vi "Test Magnet.vi"(8 "error in (no error)":errorcluster, 11 "Instrument.Cryostat in":refnum<class "Instrument.Cryostat.lvclass">) -> (0 "error out":errorcluster, 3 "Instrument.Cryostat out":refnum<class "Instrument.Cryostat.lvclass">)   [LabVIEW 2016]
uses:
  lvsrc/Instrument Types/Cryostat/Instrument.Cryostat.lvclass
  <vilib>/addons/_JKI Toolkits/Caraya/classes/Assert/Assert.lvclass
  <vilib>/addons/_JKI Toolkits/Caraya/classes/Test/Test.lvclass
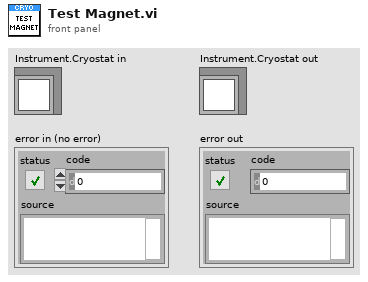
[diagram p1: front panel]
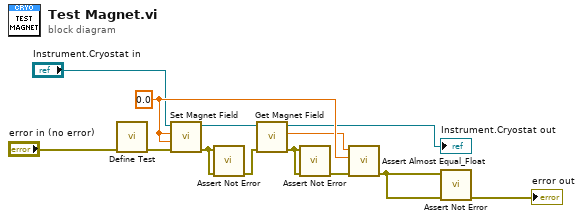
[diagram p0: block diagram]
diagram:
  w8 = 0.0 ("Angle (°)")
  n1 = call <vilib>:"Define Test.vi"("error in (no error)"="error in (no error)") -> ("error out"=w2:errorcluster)  [unwired: 10 in]
  n2 = call-dynamic "Set Magnet Field.vi"("error in (no error)"=w2, "Target Rate (T/min)"=w8, "Target Field (T)"=w8, "Instrument.Cryostat in"="Instrument.Cryostat in") -> ("error out"=w9:errorcluster, "Instrument.Cryostat out"=w6:refnum<class "Instrument.Cryostat.lvclass">)  [unwired: 6 in]
  n3 = call <vilib>:"Assert Not Error.vi"("error in (no error)"=w9, "Not Error?"=w9) -> ("error out"=w10:errorcluster)  [unwired: 9 in]
  n4 = call-dynamic "Get Magnet Field.vi"("error in (no error)"=w10, "Instrument.Cryostat in"=w6) -> ("error out"=w11:errorcluster, "B Field (T)"=w4:dbl, "Instrument.Cryostat out"=→"Instrument.Cryostat out":refnum<class "Instrument.Cryostat.lvclass">)  [unwired: 5 in, 2 out]
  n5 = call <vilib>:"Assert Not Error.vi"("error in (no error)"=w11, "Not Error?"=w11) -> ("error out"=w12:errorcluster)  [unwired: 9 in]
  n6 = call <vilib>:"Assert Almost Equal_Float.vi"("error in (no error)"=w12, "Y"=w8, "X"=w4) -> ("error out"=w13:errorcluster)  [unwired: 8 in]
  n7 = call <vilib>:"Assert Not Error.vi"("error in (no error)"=w13, "Not Error?"=w13) -> ("error out"=→"error out":errorcluster)  [unwired: 9 in]
